vi "Identify.vi"(8 "error in (no error)":errorcluster, 11 "DCLeakage in":refnum<class "DCLeakage.lvclass">=refnum) -> (0 "error out":errorcluster, 2 "Plugin is Valid":bool, 3 "DCLeakage out":refnum<class "DCLeakage.lvclass">)   [LabVIEW 2018, in "DCLeakage.lvlib" / "DCLeakage.lvclass"]
uses:
  DCLeakage.lvclass
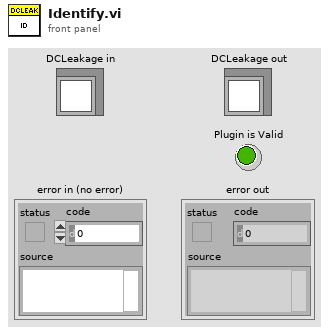
[diagram p1: front panel]
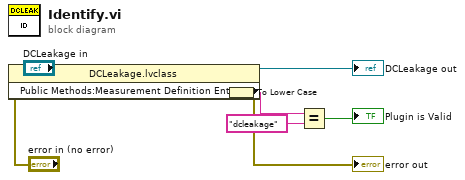
[diagram p0: block diagram]
diagram:
  n1 = property class="DCLeakage.lvclass"(reference="DCLeakage in", error in="error in (no error)") -> (reference out=→"DCLeakage out":refnum<class "DCLeakage.lvclass">, error out=→"error out":errorcluster, "Public Methods:Measurement Definition Entry"=w4)
  n2 = To Lower Case(string=w4) -> (all lower case string=w2:string)
  n3 = Equal?(x=w2, y="dcleakage") -> (x = y?=→"Plugin is Valid":bool)
